vi "exercise example 2.vi"() -> ()   [LabVIEW 2021]
panel:
  in  "Numeric 4":i32=10
  out "x+ 1":dbl
  in  "x":dbl
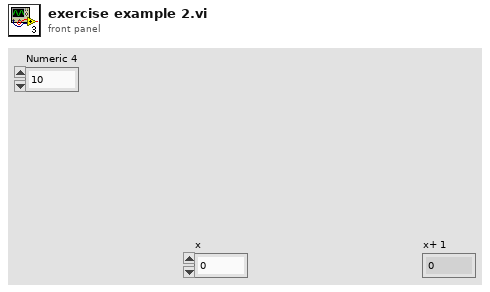
[diagram p1: front panel]
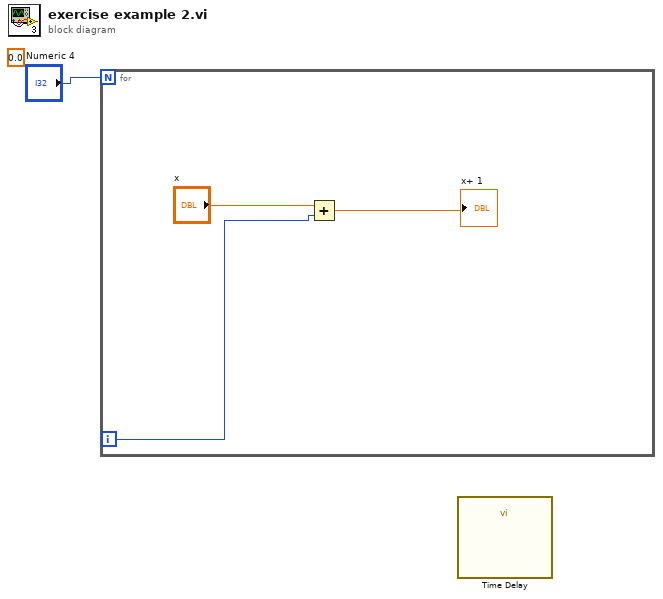
[diagram p0: block diagram]
diagram:
  (unwired) 0.0 ("Numeric 3")
  n1 = for {
    N: "Numeric 4" -> [_]
    i -> [w2]
    n2 = Add(x="x", y=w2) -> (x+y=→"x+ 1":dbl)
  }
  n3 = call "Time Delay"() -> ()  [unwired: 11 in, 1 out]
